vi "SetArmCount.vi"(8 "Error In":errorcluster, 9 "Infinite?":bool, 10 "Count (1-3000)":u16=1 min=1 max=3000 step=1, 11 "Keithley 6485 In":refnum<visa-resource-name>) -> (0 "Error Out":errorcluster, 3 "Keithley 6485 Out":refnum<visa-resource-name>)   [LabVIEW 2012, in "Keithley-6485.lvlib"]
uses:
  Keithley-6485.lvlib
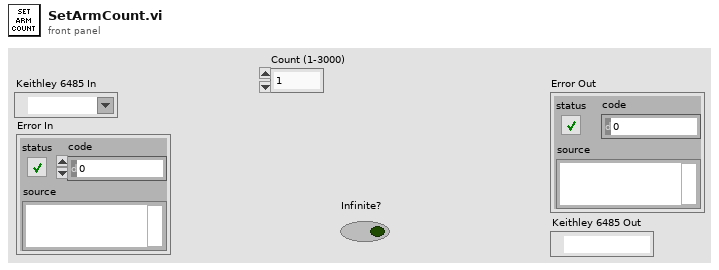
[diagram p1: front panel]
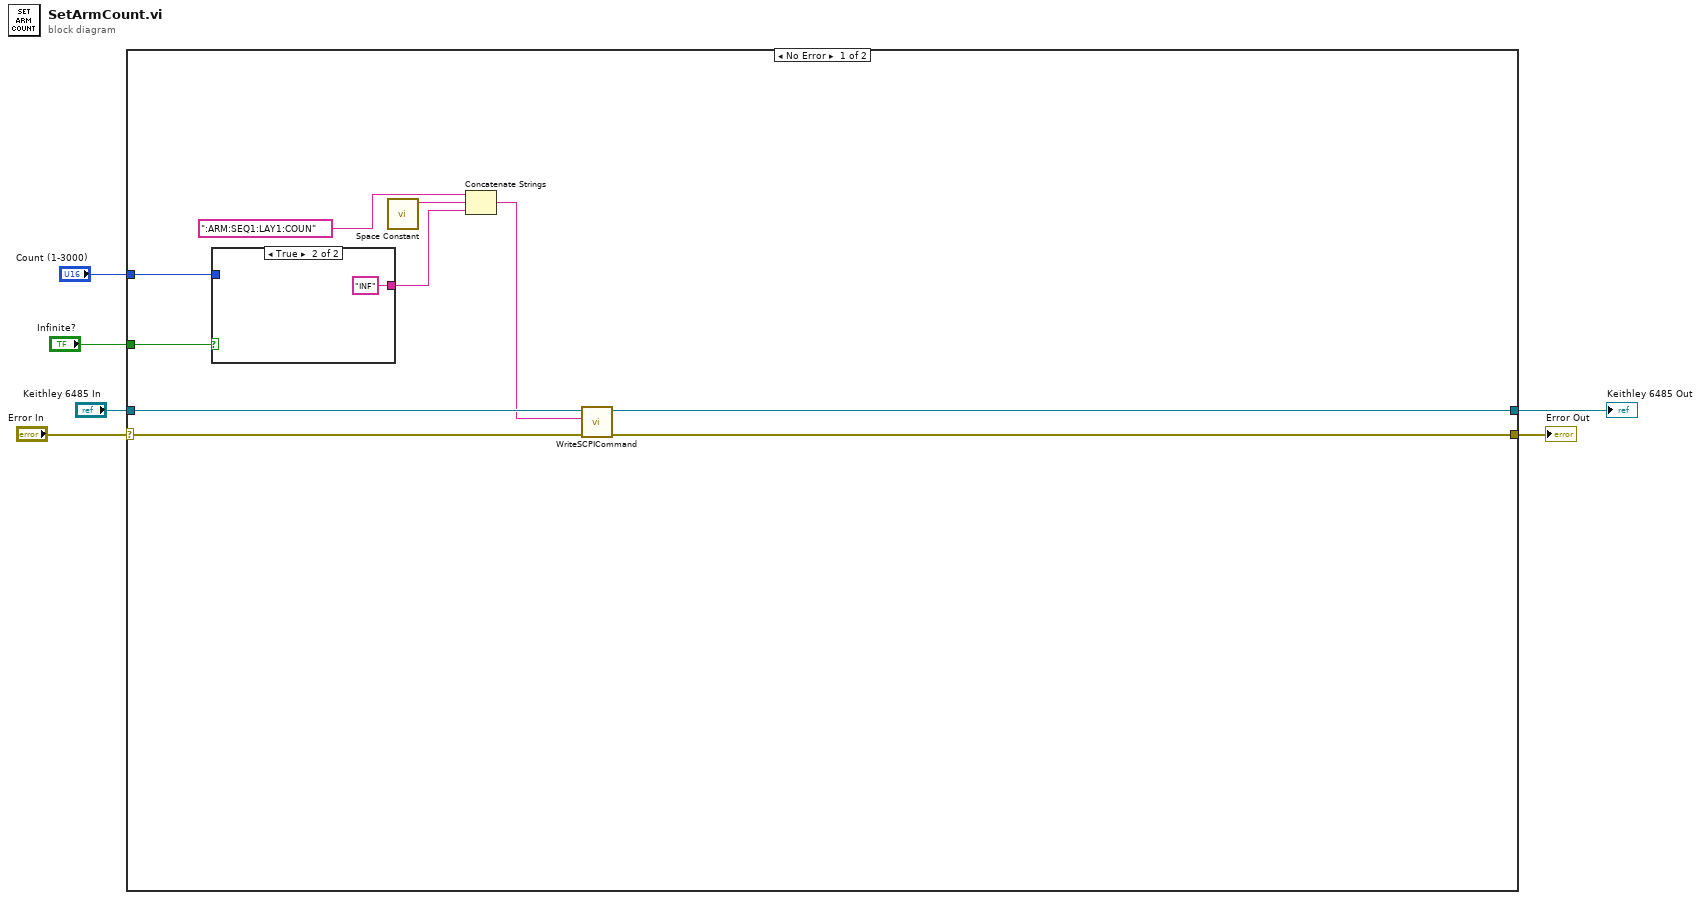
[diagram p0: block diagram]
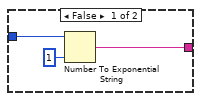
[diagram p2: hidden frame]
diagram:
  n1 = case shown="No Error" "Error In" {
    selector: "Error In" -> [w16 w21]
    tunnel: "Keithley 6485 In" -> [w15 w22]
    tunnel: [w8 w21] -> w4
    tunnel: [w9 w22] -> w3
    tunnel: "Count (1-3000)" -> [w12 _]
    tunnel: "Infinite?" -> [w7 _]
    frame No Error {
      n2 = case shown="True" w7 {
        tunnel: w12 -> [w19 _]
        tunnel: [w17 "INF"] -> w11
        frame False {
          n3 = Number To Exponential String(number=w19, precision (6)=i16 1) -> (E-format string=w17:string)  [unwired: 2 in]
        }
        frame True {
        }
      }
      n4 = call <vilib>:"Space Constant.vi"() -> ("String"=w13:string)
      n5 = Concatenate Strings(":ARM:SEQ1:LAY1:COUN" ("string"), w13, w11) -> (w10:string)
      n6 = call "WriteSCPICommand.vi"("Error In"=w16, "SCPI Command"=w10, "Keithley 6482 In"=w15) -> ("Error Out"=w8:errorcluster, "Keithley 6482 Out"=w9:refnum<visa-resource-name>)  [unwired: 7 in]
    }
    frame Error {
    }
  }
  "Error Out" <- w4
  "Keithley 6485 Out" <- w3
